vi "Test_DSP1500-30WE_3icon.vi"() -> ()   [LabVIEW 2019]
uses:
  _ctrl/DSP_config.ctl
  _ctrl/DSP_action.ctl
  _ctrl/rw.ctl
panel:
  out "error out":errorcluster
  in  "config":T1={"Port"="TCPIP0::192.168.0.14::HISLIP0::INSTR", "OVP Level"=0.0, "OCP Level"=0.0, "Current"=0.0, "Voltage"=0.0} {"OCP Level" format="%#_13g"; "OVP Level" format="%#_13g"}
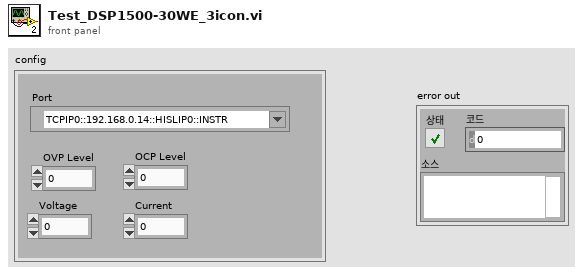
[diagram p1: front panel]
types:
  T1 = typedef "DSP_config.ctl" = cluster{"Port":refnum<visa-resource-name>, "OVP Level":dbl, "OCP Level":dbl, "Current":dbl, "Voltage":dbl}
  T2 = typedef "DSP_action.ctl" = enum16{"False", "cont", "on", "off", "discont", "protection", "preread", "level", "read", "stop", "exit"}
  T3 = typedef "rw.ctl" = enum16{"read", "write"}
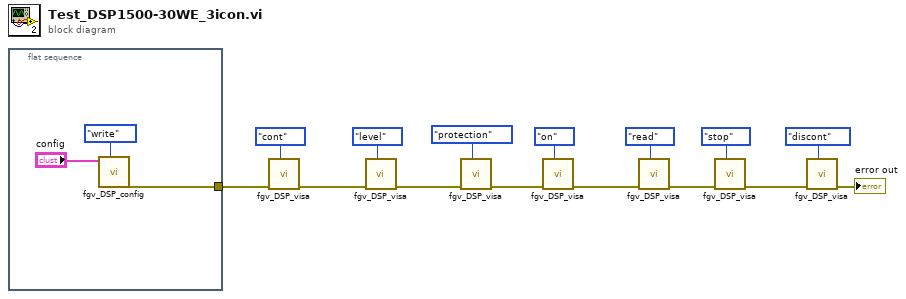
[diagram p0: block diagram]
diagram:
  n1 = flat-sequence {
    tunnel: [w16] -> w14
    frame #0 {
      n2 = call "fgv_DSP_config.vi"("cmd"=rw."write", "DSP1950 Config"="config") -> ("error out"=w16:errorcluster)  [unwired: 8 in, 1 out]
    }
  }
  n3 = call "fgv_DSP_visa.vi"("action"=DSP_action."cont", "error in"=w14) -> ("error out"=w8:errorcluster)  [unwired: 9 in]
  n4 = call "fgv_DSP_visa.vi"("action"=DSP_action."level", "error in"=w8) -> ("error out"=w7:errorcluster)  [unwired: 9 in]
  n5 = call "fgv_DSP_visa.vi"("action"=DSP_action."protection", "error in"=w7) -> ("error out"=w3:errorcluster)  [unwired: 9 in]
  n6 = call "fgv_DSP_visa.vi"("action"=DSP_action."on", "error in"=w3) -> ("error out"=w2:errorcluster)  [unwired: 9 in]
  n7 = call "fgv_DSP_visa.vi"("action"=DSP_action."read", "error in"=w2) -> ("error out"=w6:errorcluster)  [unwired: 9 in]
  n8 = call "fgv_DSP_visa.vi"("action"=DSP_action."stop", "error in"=w6) -> ("error out"=w5:errorcluster)  [unwired: 9 in]
  n9 = call "fgv_DSP_visa.vi"("action"=DSP_action."discont", "error in"=w5) -> ("error out"=→"error out":errorcluster)  [unwired: 9 in]
